vi "Channel Status.vi"(5 "All Channels (T)":bool=TRUE, 7 "Channel":u8, 8 "error in (no error)":errorcluster, 11 "BoardHandle":T2) -> (0 "error out":errorcluster, 2 "Channel Status Array":T1(array[cluster]), 3 "BoardHandle out":T2)   [LabVIEW 2018, in "CAEN PSM.lvlib"]
doc: "Returns status for channels or a desired channel."
uses:
  <instrlib>/CAEN PSM/CAEN PSM.lvlib
  <instrlib>/CAEN PSM/Private/BoardHandle.ctl
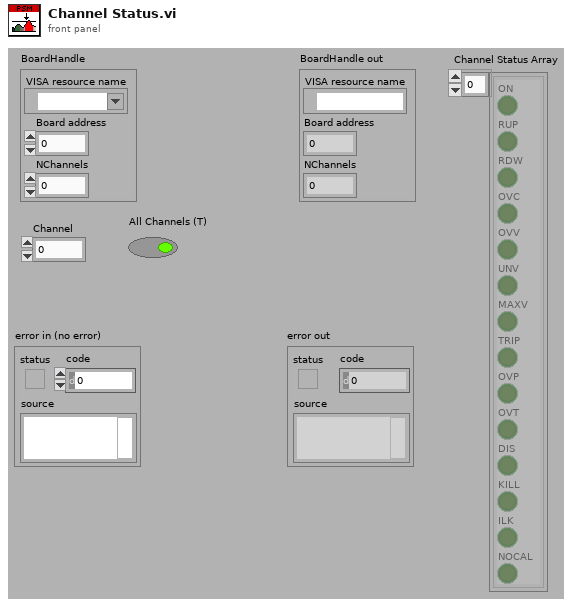
[diagram p1: front panel]
types:
  T1 = cluster{"ON":bool, "RUP":bool, "RDW":bool, "OVC":bool, "OVV":bool, "UNV":bool, "MAXV":bool, "TRIP":bool, "OVP":bool, "OVT":bool, "DIS":bool, "KILL":bool, "ILK":bool, "NOCAL":bool}[]
  T2 = typedef "CAEN PSM.lvlib/BoardHandle.ctl" = cluster{"VISA resource name":refnum<visa-resource-name>, "Board address":u8, "NChannels":u8}
  T3 = cluster{"OVV":bool, "UNV":bool, "MAXV":bool, "TRIP":bool, "OVP":bool, "OVT":bool, "DIS":bool, "KILL":bool, "ILK":bool, "OVC":bool, "RDW":bool, "RUP":bool, "ON":bool, "NOCAL":bool}[]
  T4 = cluster{"Boolean array[0]":bool, "Boolean array[1]":bool, "Boolean array[2]":bool, "Boolean array[3]":bool, "Boolean array[4]":bool, "Boolean array[5]":bool, "Boolean array[6]":bool, "Boolean array[7]":bool, "Boolean array[8]":bool, "Boolean array[9]":bool, "Boolean array[10]":bool, "Boolean array[11]":bool, "Boolean array[12]":bool, "Boolean array[13]":bool}
  T5 = cluster{"Boolean array[0]":bool, "Boolean array[1]":bool, "Boolean array[2]":bool, "Boolean array[3]":bool, "Boolean array[4]":bool, "Boolean array[5]":bool, "Boolean array[6]":bool, "Boolean array[7]":bool, "Boolean array[8]":bool, "Boolean array[9]":bool, "Boolean array[10]":bool, "Boolean array[11]":bool, "Boolean array[12]":bool, "Boolean array[13]":bool}[]
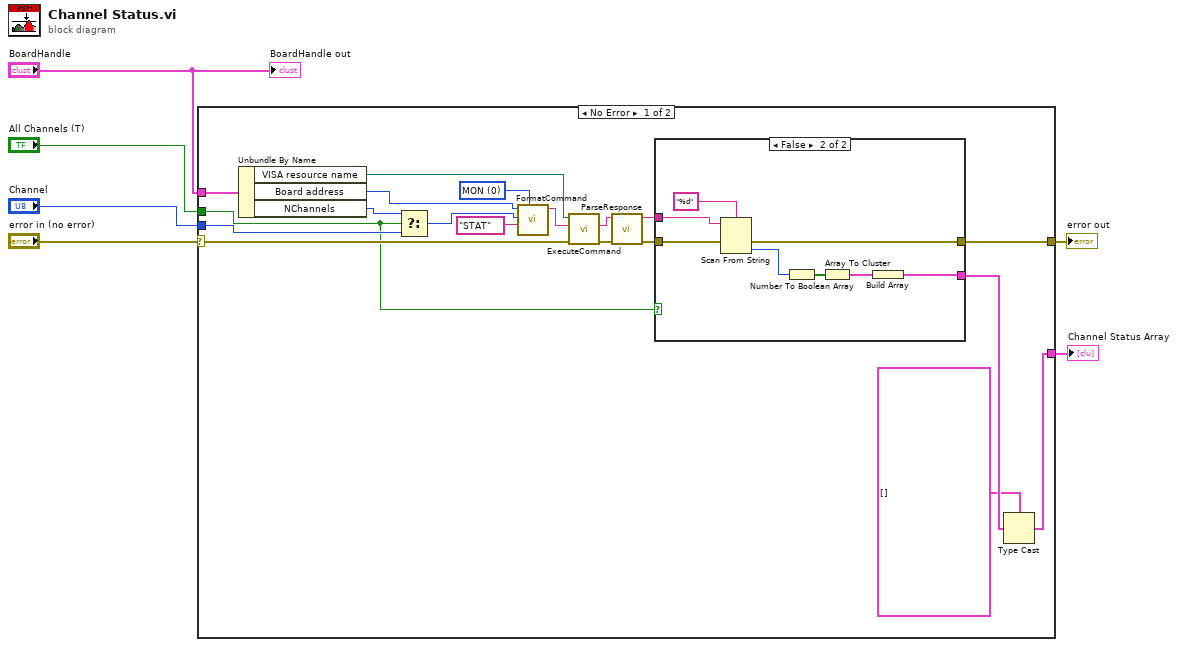
[diagram p0: block diagram]
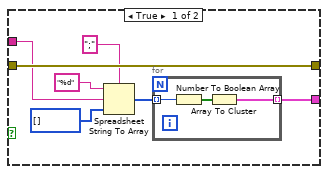
[diagram p2: hidden frame]
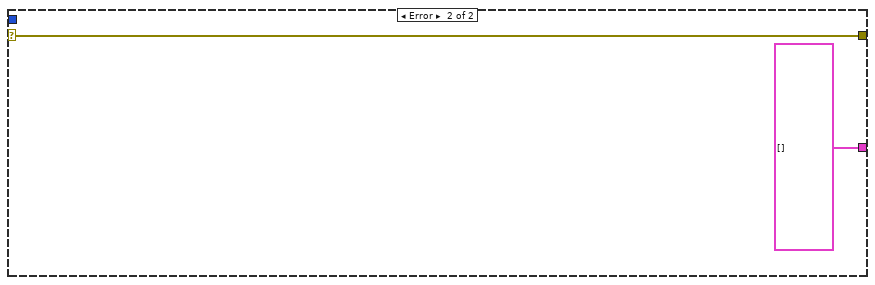
[diagram p3: hidden frame]
diagram:
  n1 = case shown="No Error" "error in (no error)" {
    selector: "error in (no error)" -> [w16 w45]
    tunnel: "All Channels (T)" -> [w7 _]
    tunnel: "Channel" -> [w23 _]
    tunnel: [w8 w45] -> w3
    tunnel: "BoardHandle" -> [w17 _]
    tunnel: [w9 T3 []] -> w1
    frame No Error {
      w24 = u8 0 items=["MON", "SET"] ("CMD")
      n2 = Unbundle By Name(w17) -> ("VISA resource name"=w21:refnum<visa-resource-name>, "Board address"=w25:u8, "NChannels"=w13:u8)
      n3 = Select(t=w13, s=w7, f=w23) -> (s? t:f=w22:u8)
      n4 = call <instrlib>:"FormatCommand.vi"("CMD (MON)"=w24, "PAR"="STAT", "CH"=w22, "BD (0)"=w25) -> ("cmd"=w20:string)  [unwired: 7 in]
      n5 = call <instrlib>:"ExecuteCommand.vi"("error in (no error)"=w16, "Command"=w20, "VISA resource name"=w21) -> ("error out"=w19:errorcluster, "Response"=w18:string)  [unwired: 6 in, 1 out]
      n6 = call <instrlib>:"ParseResponse.vi"("error in (no error)"=w19, "Response"=w18) -> ("error out"=w12:errorcluster, "val"=w14:string)  [unwired: 6 in, 2 out]
      n7 = case shown="False" w7 {
        tunnel: w14 -> [w30 w43]
        tunnel: w12 -> [w32 w41]
        tunnel: [w26 w36] -> w11
        tunnel: [w32 w38] -> w8
        frame True {
          n8 = Spreadsheet String To Array(delimiter (Tab)=";", format string="%d", spreadsheet string=w30, array type (2D Dbl)=i32[] []) -> (array=w27:i32[])
          n9 = for {
            tunnel: w27 -> [w34] mode=indexing
            tunnel: [w33] -> w26 mode=indexing
            n10 = Number To Boolean Array(number=w34) -> (Boolean array=w35:bool[])
            n11 = Array To Cluster(array=w35) -> (cluster=w33:T4)
          }
        }
        frame False {
          n12 = Scan From String(format string="%d", input string=w43, error in=w41) -> (error out=w38:errorcluster, output 1=w40:i32)  [unwired: 2 in, 2 out]
          n13 = Number To Boolean Array(number=w40) -> (Boolean array=w39:bool[])
          n14 = Array To Cluster(array=w39) -> (cluster=w37:T4)
          n15 = Build Array(w37) -> (w36:T5)
        }
      }
      n16 = Type Cast(type=T1 [], x=w11) -> (*(type *) &x=w9:T1)
    }
    frame Error {
    }
  }
  "error out" <- w3
  "Channel Status Array" <- w1
  "BoardHandle out" <- "BoardHandle"
